vi "Wait for Distributed Manager.vi"(8 "error in (no error)":errorcluster, 11 "Error Manager in":refnum<class "Local Error Manager.lvclass">) -> (0 "error out":errorcluster, 3 "Error Manager out":refnum<class "Local Error Manager.lvclass">)   [LabVIEW 2020, in "TALOS.lvlib" / "Error Manager.lvlib" / "Local Error Manager.lvclass"]
uses:
  Local Error Manager.lvclass
  C:/LabVIEW Code/TALOS/talos/Internal uServices/System uServices/Error Manager/Error Manager.lvclass
  Ancestor/Ancestor/Infinite Message Selector.ctl
  Error Manager Consumer Case Selector.ctl
  Error Manager.lvclass/Error Manager.ctl
  Write Distributed Error Manager Started flag.vi
  Read Distributed flag.vi
  Support VIs/Global Memory.vi
  Local Error Manager.lvclass/Local Error Manager.ctl
  Ancestor/Ancestor/Ancestor.lvclass
  Error Manager.lvclass
  TALOS.lvlib
  C:/LabVIEW Code/TALOS/talos/Father of all uServices/Father of all uServices/Father of all uServices.lvclass
  C:/LabVIEW Code/TALOS/talos/Ancestor/Ancestor/Ancestor.lvclass
  C:/LabVIEW Code/TALOS/builds/Actor Framework PPL/Actor Framework.lvlibp/1abvi3w/vi.lib/ActorFramework/Actor/Actor.lvclass
  C:/LabVIEW Code/TALOS/talos/Internal uServices/System uServices/Error Manager/Local Error Manager/Local Error Manager.lvclass
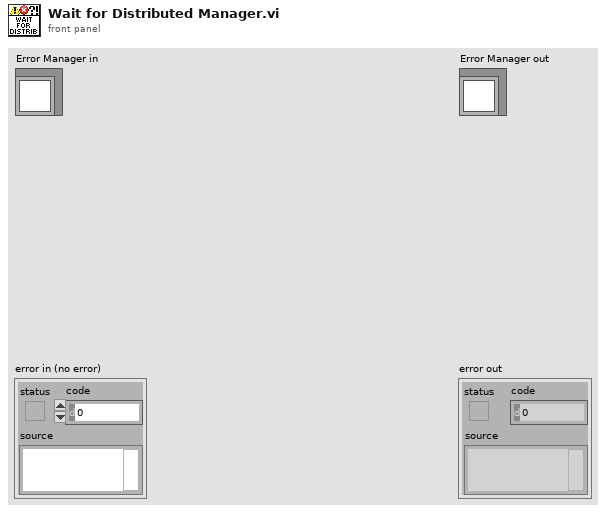
[diagram p1: front panel]
types:
  T1 = typedef "TALOS.lvlib/Error Manager.lvlib/Error Manager.lvclass/Error Manager Consumer Case Selector.ctl" = enum16{"Digest Error", "Dismiss Error", "Dismiss All", "Show Error Details", "Filter out Errors", "Clear Filters", "Check Distributed Error Manager"}
  T2 = typedef "TALOS.lvlib/Ancestor.lvlib/Ancestor.lvclass/Infinite Message Selector.ctl" = enum16{"Start", "Stop", "Check", "Flush (Stop all)", "Init"}
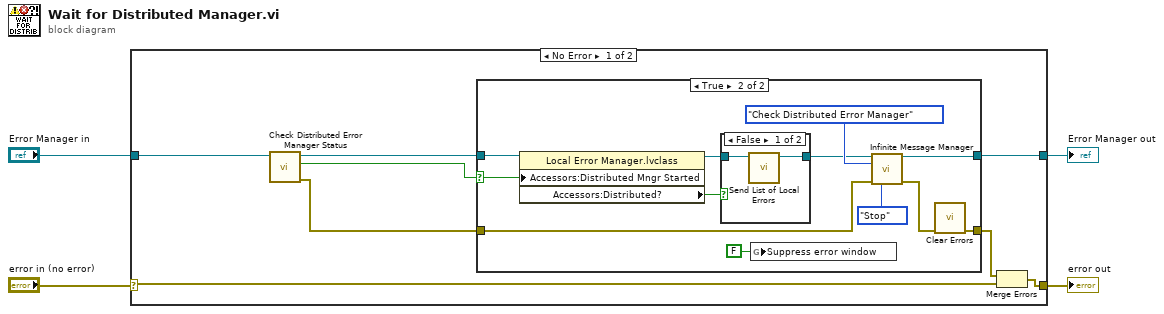
[diagram p0: block diagram]
diagram:
  n1 = case shown="No Error" "error in (no error)" {
    selector: "error in (no error)" -> [w10 w31]
    tunnel: [w8 w31] -> w3
    tunnel: [w12 w30] -> w1
    tunnel: "Error Manager in" -> [w7 w30]
    frame No Error {
      n2 = call "Check Distributed Error Manager Status.vi"("Local Error Manager in"=w7) -> ("error out"=w11:errorcluster, "uService found?"=w5:bool, "Local Error Manager out"=w6:refnum<class "Local Error Manager.lvclass">)  [unwired: 8 in]
      n3 = case shown="True" w5 {
        selector: w5 -> [_ w25]
        tunnel: w6 -> [w14 w26]
        tunnel: [w14 w18] -> w12
        tunnel: w11 -> [w13 w20]
        tunnel: [w13 w16] -> w9
        frame False {
        }
        frame True {
          n4 = property class="Local Error Manager.lvclass"(reference=w26, "Accessors:Distributed Mngr Started"=w25) -> (reference out=w24:refnum<class "Local Error Manager.lvclass">, "Accessors:Distributed?"=w23:bool)  [unwired: 1 in, 1 out]
          n5 = case shown="False" w23 {
            tunnel: w24 -> [w28 w29]
            tunnel: [w27 w29] -> w19
            frame False {
              n6 = call "Send List of Local Errors.vi"("Local Error Manager in"=w28) -> ("Local Error Manager out"=w27:refnum<class "Local Error Manager.lvclass">)  [unwired: 9 in, 1 out]
            }
            frame True {
            }
          }
          n7 = global write "Global Memory.vi" "Suppress error window"(FALSE ("Suppress error window")) -> ()
          n8 = call-dynamic "Infinite Message Manager.vi"("Father of all uServices in"=w19, "Consumer Case Selector"=Error_Manager_Consumer_Case_Selector."Check Distributed Error Manager" ("ErrMgr Case Selector"), "error in (no error)"=w20, "Infinite Message Selector"=Infinite_Message_Selector."Stop") -> ("Father of all uServices out"=w18:refnum<class "Local Error Manager.lvclass">, "error out"=w17:errorcluster)  [unwired: 9 in, 1 out]
          n9 = call <vilib>:"Clear Errors.vi"("error in (no error)"=w17) -> ("error out"=w16:errorcluster)  [unwired: 5 in, 1 out]
        }
      }
      n10 = Merge Errors(w9, w10) -> (w8:errorcluster)
    }
    frame Error {
    }
  }
  "error out" <- w3
  "Error Manager out" <- w1
